vi "Get Mapping Targets.vi"(8 "error in (no error)":errorcluster, 11 "PDO Mapping in":refnum<class "PDO Mapping.lvclass">) -> (0 "error out":errorcluster, 2 "Mapping Targets":refnum<class "OD Entry.lvclass">[](array[class]), 3 "PDO Mapping out":refnum<class "PDO Mapping.lvclass">)   [LabVIEW 2019, in "PDO Grid.lvlib" / "PDO Mapping.lvclass"]
uses:
  PDO Mapping.lvclass
  Core/OD Entry/OD Entry.lvclass
  PDO Mapping.lvclass/PDO Mapping.ctl
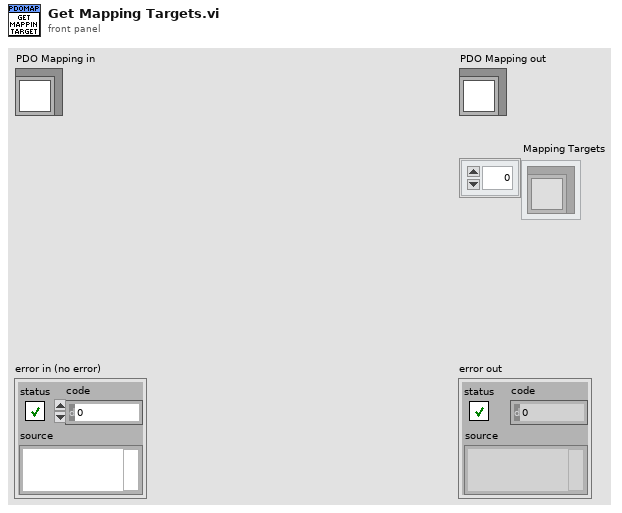
[diagram p1: front panel]
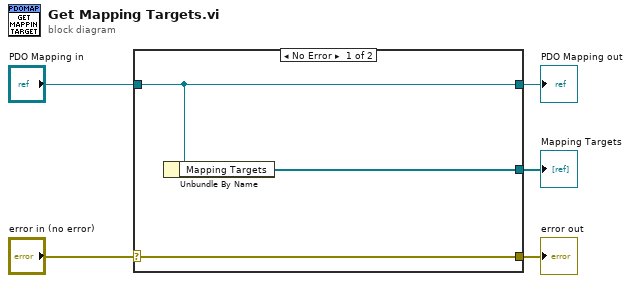
[diagram p0: block diagram]
diagram:
  n1 = case shown="No Error" "error in (no error)" {
    selector: "error in (no error)" -> [w8 w9]
    tunnel: [w8 w9] -> w4
    tunnel: [w7 w10] -> w2
    tunnel: "PDO Mapping in" -> [w7 w10]
    tunnel: [w6 _] -> w1
    frame No Error {
      n2 = Unbundle By Name(w7) -> ("Mapping Targets"=w6:refnum<class "OD Entry.lvclass">[])
    }
    frame Error {
    }
  }
  "error out" <- w4
  "PDO Mapping out" <- w2
  "Mapping Targets" <- w1
